vi "Clean image graph.vi"(8 "error in (no error)":errorcluster, 11 "CCD in":refnum<class "CCD.lvclass">) -> (0 "error out":errorcluster, 3 "CCD out":refnum<class "CCD.lvclass">)   [LabVIEW 2018, in "CCD.lvclass"]
uses:
  CCD.lvclass
  CCD.lvclass/CCD.ctl
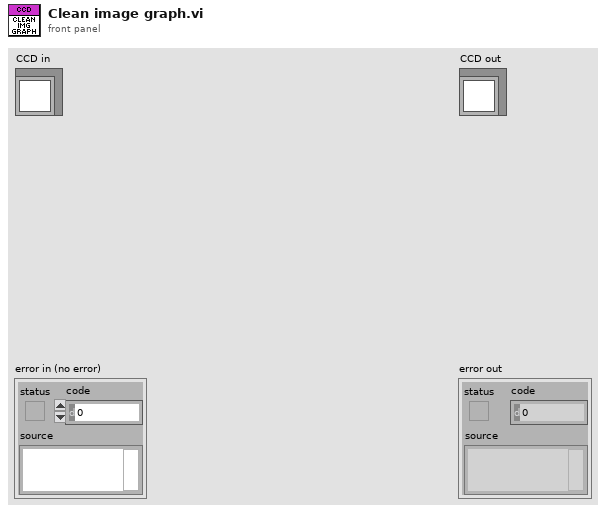
[diagram p1: front panel]
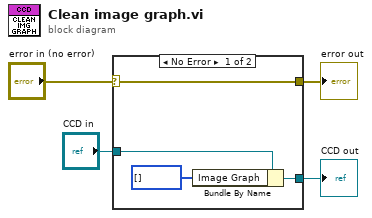
[diagram p0: block diagram]
diagram:
  n1 = case shown="No Error" "error in (no error)" {
    selector: "error in (no error)" -> [w8 w10]
    tunnel: [w8 w10] -> w1
    tunnel: [w6 w9] -> w2
    tunnel: "CCD in" -> [w7 w9]
    frame No Error {
      n2 = Bundle By Name(cluster=w7, "Image Graph"=i32[] []) -> (w6:refnum<class "CCD.lvclass">)
    }
    frame Error {
    }
  }
  "error out" <- w1
  "CCD out" <- w2
